vi "h5_save_stats.vi"(4 "stats":T1[](array[typedef])=[{"min"=0.0, "t_min"=0.0, "max"=0.0, "t_max"=0.0, "range"=0.0, "mean"=0.0, "stdev"=0.0}, {"min"=-0.5, "t_min"=3.72e-06, "max"=0.5, "t_max"=4.38e-07, "range"=1.0, "mean"=0.021804704021121078, "stdev"=0.4509986732980552}], 7 "TYPE":string="STAT_#", 9 "record stats.":bool[](array[boolean])=[FALSE, FALSE], 10 "SQUID":string="100", 11 "H5":path[](array[path])=[path ""]) -> (0 "error out":errorcluster)   [LabVIEW 2015, in "oscilloscope.lvlib"]
uses:
  oscilloscope.lvlib
  osc_stats.ctl
  <vilib>/UPVI/lvhdf5/dataset.llb/LVH5D Operation.ctl
  <vilib>/UPVI/lvhdf5/dataset.llb/Simple OpenCreateReplace Dataset (Variant).vi
  <vilib>/UPVI/lvhdf5/dataset.llb/H5Dwrite (Variant).vi
  <vilib>/UPVI/lvhdf5/dataset.llb/Append Element(s) to Dataset (Variant).vi
  <vilib>/UPVI/lvhdf5/dataset.llb/Simple OpenCreateReplace Dataset.xnode
  <vilib>/UPVI/lvhdf5/library.llb/HDF5 Ref.ctl
  <vilib>/UPVI/lvhdf5/dataset.llb/H5Dwrite.xnode
  <vilib>/UPVI/lvhdf5/dataset.llb/Append Element(s) to Dataset.xnode
  oskar_tools/oskar_tools.lvlib
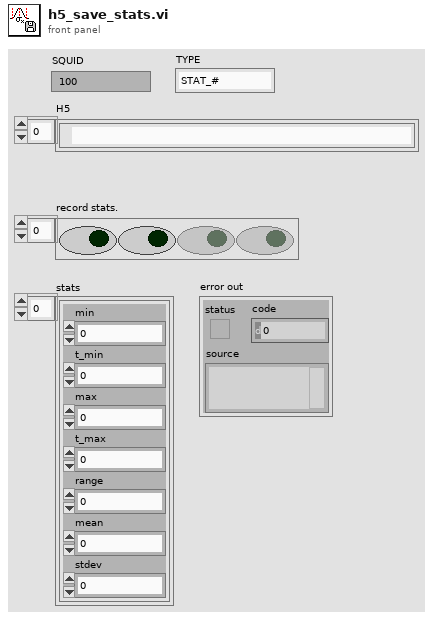
[diagram p1: front panel]
types:
  T1 = typedef "oscilloscope.lvlib/osc_stats.ctl" = cluster{"min":dbl, "t_min":dbl, "max":dbl, "t_max":dbl, "range":dbl, "mean":dbl, "stdev":dbl}
  T2 = typedef "Semaphore RefNum" = refnum<k1>
  T3 = typedef "LVH5D Operation.ctl" = enum16{"open", "replace", "create", "open or create", "create or replace", "create or replace with confirmation"}
  T4 = typedef "HDF5 Ref.ctl" = refnum<k1>
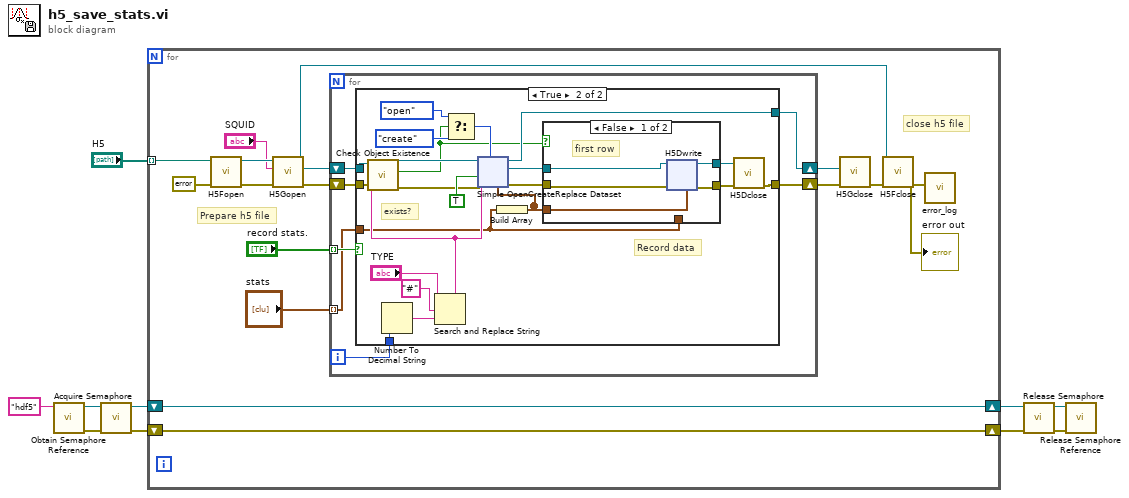
[diagram p0: block diagram]
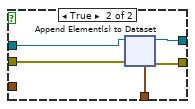
[diagram p3: hidden frame]
diagram:
  n1 = call <vilib>:"Obtain Semaphore Reference.vi"("name (unnamed)"="hdf5") -> ("error out"=w8:errorcluster, "semaphore"=w9:T2)  [unwired: 4 in, 1 out]
  n2 = call <vilib>:"Acquire Semaphore.vi"("error in (no error)"=w8, "semaphore"=w9) -> ("error out"=w3:errorcluster, "semaphore out"=w4:T2)  [unwired: 3 in, 1 out]
  n3 = for {
    tunnel: "H5" -> [w24] mode=indexing
    shift-right: [w25] -> w2
    shift-left: w4 -> [w25]
    shift-right: [w26] -> w1
    shift-left: w3 -> [w26]
    # "close h5 file"
    # "Prepare h5 file"
    n4 = call <vilib>:"H5Fopen.vi"("error in (no error)"=errorcluster {"status"=FALSE, "code"=0, "source"=""} ("error out"), "path"=w24) -> ("error out"=w22:errorcluster, "HDF5 Ref out"=w21:T4)  [unwired: 6 in]
    n5 = call <vilib>:"H5Gopen.vi"("error in (no error)"=w22, "Name"="SQUID", "HDF5 Ref"=w21) -> ("error out"=w16:errorcluster, "HDF5 Group Ref"=w17:T4, "HDF5 Ref out"=w19:T4)  [unwired: 4 in]
    n6 = for {
      shift-right: [w27] -> w14
      shift-left: w17 -> [w31]
      shift-right: [w33] -> w15
      shift-left: w16 -> [w30]
      tunnel: "record stats." -> [w29] mode=indexing
      tunnel: "stats" -> [w28] mode=indexing
      i -> [w32]
      n7 = case shown="True" w29 {
        tunnel: [w35 w56] -> w33
        tunnel: [w34 w55] -> w27
        tunnel: w32 -> [_ w51]
        tunnel: w31 -> [w34 w50]
        tunnel: w30 -> [w35 w48]
        tunnel: w28 -> [_ w36]
        frame False {
        }
        frame True {
          # "exists?"
          # "Record data"
          n8 = Number To Decimal String(number=w51) -> (decimal integer string=w54:string)  [unwired: 1 in]
          n9 = Search and Replace String(input string="TYPE", search string="#", replace string=w54) -> (result string=w49:string)  [unwired: 5 in, 3 out]
          n10 = call <vilib>:"Check Object Existence.vi"("error in (no error)"=w48, "name"=w49, "HDF5 Ref"=w50) -> ("error out"=w47:errorcluster, "Exists"=w41:bool, "HDF5 Ref out"=w46:T4)  [unwired: 4 in]
          n11 = Select(t=LVH5D_Operation."open" ("operation"), s=w41, f=LVH5D_Operation."create" ("operation")) -> (s? t:f=w43:T3)
          n12 = Build Array(w36) -> (w39:T1[])
          n13 = xnode "Simple OpenCreateReplace Dataset"("Dataset Path"=w49, "HDF5 Ref"=w46, "Unlimited  dataset (F)"=TRUE, "error in (no error)"=w47, "operation"=w43, "Datatype and Dataspace"=w39) -> ("HDF5 Dataset Ref out"=w40:T4, "HDF5 Ref out"=w55:T4, "error out"=w42:errorcluster)  [unwired: 2 in]
          n14 = case shown="False" w41 {
            tunnel: w42 -> [w62 w73]
            tunnel: [w61 w76] -> w37
            tunnel: [w60 w75] -> w38
            tunnel: w40 -> [w59 w72]
            tunnel: w39 -> [w58 _]
            tunnel: w36 -> [_ w74]
            frame False {
              # "first row"
              n15 = xnode "H5Dwrite"("HDF5 Dataset Ref"=w59, "error in (no error)"=w62, "Data"=w58) -> ("HDF5 Ref out"=w60:T4, "error out"=w61:errorcluster)  [unwired: 4 in]
            }
            frame True {
              n16 = xnode "Append Element(s) to Dataset"("HDF5 Dataset Ref"=w72, "error in (no error)"=w73, "Data Element(s)"=w74) -> ("HDF5 Dataset out"=w75:T4, "error out"=w76:errorcluster)  [unwired: 1 in, 2 out]
            }
          }
          n17 = call <vilib>:"H5Dclose.vi"("error in (no error)"=w37, "HDF5 Dataset Ref"=w38) -> ("error out"=w56:errorcluster)  [unwired: 7 in]
        }
      }
    }
    n18 = call <vilib>:"H5Gclose.vi"("error in (no error)"=w15, "HDF5 Group Ref"=w14) -> ("error out"=w20:errorcluster)  [unwired: 7 in]
    n19 = call <vilib>:"H5Fclose.vi"("error in (no error)"=w20, "HDF5 Ref"=w19) -> ("error out"=w18:errorcluster)  [unwired: 7 in]
    "error out" <- w18
    n20 = call "error_log.vi"("error"=w18) -> ()  [unwired: 10 in]
  }
  n21 = call <vilib>:"Release Semaphore.vi"("error in (no error)"=w1, "semaphore"=w2) -> ("error out"=w6:errorcluster, "semaphore out"=w5:T2)  [unwired: 4 in]
  n22 = call <vilib>:"Release Semaphore Reference.vi"("error in (no error)"=w6, "semaphore"=w5) -> ()  [unwired: 8 in, 2 out]
